vi "E New.vi"(0 "model Path/模板路径":path, 1 "Visible/表格可见？(False)":bool, 11 "Error In (no error)":errorcluster) -> (4 "Excel._Application":refnum<k7>, 6 "Excel._Workbook":refnum<k7>, 15 "Error Out":errorcluster)   [LabVIEW 2014]
doc: "打开指定路径下指定名称的电子表格，可以设置表格的可见或不可见。"
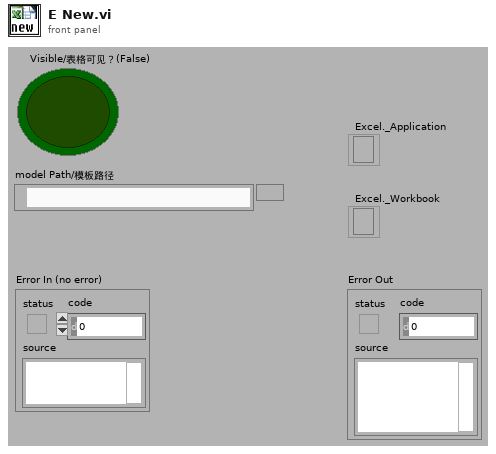
[diagram p1: front panel]
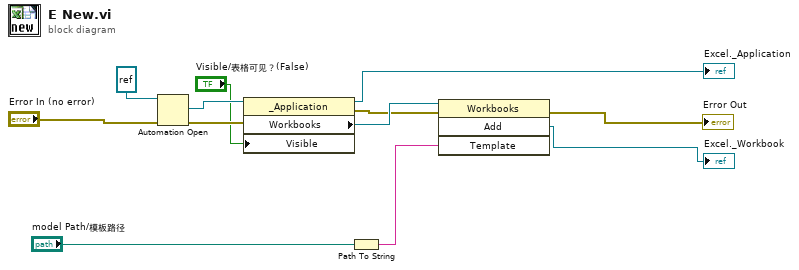
[diagram p0: block diagram]
diagram:
  n1 = Automation Open(error in (no error)="Error In (no error)", Automation Refnum=refnum<k7> refnum ("Excel._Application")) -> (Automation Refnum=w12:refnum<k7>, error out=w10:errorcluster)  [unwired: 2 out]
  n2 = property class="_Application"(reference=w12, error in=w10, "Visible"="Visible/表格可见？(False)") -> (reference out=→"Excel._Application":refnum<k7>, error out=w8:errorcluster, "Workbooks"=w11:refnum<k7>)
  n3 = Path To String(path="model Path/模板路径") -> (string=w7:string)
  n4 = invoke class="Workbooks" method="Add"(reference=w11, error in=w8, "Template"=w7) -> (error out=→"Error Out":errorcluster, "Add"=→"Excel._Workbook":refnum<k7>)  [unwired: 1 in, 2 out]
